vi "WriteMasterData.vi"(8 "error in (no error)":errorcluster, 10 "New data":u8[](array[numeric]), 11 "Array in":refnum<vi>) -> (0 "error out":errorcluster)   [LabVIEW 2016]
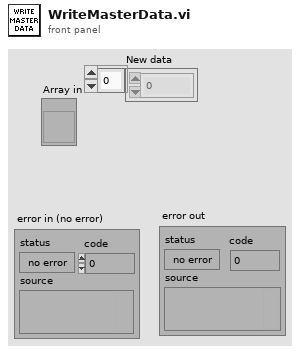
[diagram p1: front panel]
types:
  T1 = typedef "Semaphore RefNum" = refnum<k1>
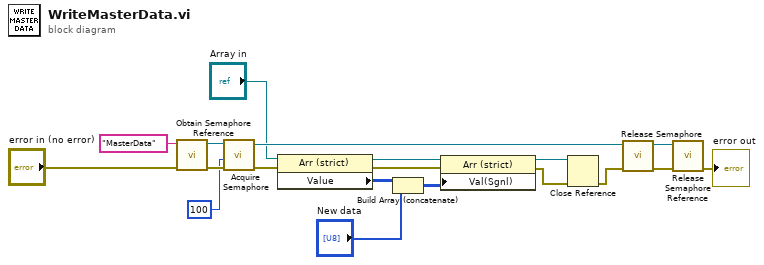
[diagram p0: block diagram]
diagram:
  n1 = call <vilib>:"Obtain Semaphore Reference.vi"("error in (no error)"="error in (no error)", "name (unnamed)"="MasterData") -> ("error out"=w6:errorcluster, "semaphore"=w7:T1)  [unwired: 3 in, 1 out]
  n2 = call <vilib>:"Acquire Semaphore.vi"("error in (no error)"=w6, "ms timeout (-1)"=100, "semaphore"=w7) -> ("error out"=w8:errorcluster, "semaphore out"=w14:T1)  [unwired: 2 in, 1 out]
  n3 = property on="Property Node" class="Arr (strict)"(reference="Array in", error in=w8) -> (reference out=w10:refnum<vi>, error out=w11:errorcluster, "Value"=w12:u8[][])
  n4 = Build Array (concatenate)(w12, "New data") -> (w13:u8[][])
  n5 = property on="Property Node" class="Arr (strict)"(reference=w10, error in=w11, "Val(Sgnl)"=w13) -> (reference out=w16:refnum<vi>, error out=w15:errorcluster)
  n6 = Close Reference(reference=w16, error in (no error)=w15) -> (error out=w17:errorcluster)
  n7 = call <vilib>:"Release Semaphore.vi"("error in (no error)"=w17, "semaphore"=w14) -> ("error out"=w18:errorcluster, "semaphore out"=w19:T1)  [unwired: 4 in]
  n8 = call <vilib>:"Release Semaphore Reference.vi"("error in (no error)"=w18, "semaphore"=w19) -> ("error out"=→"error out":errorcluster)  [unwired: 8 in, 1 out]
